vi "VI Stoermeldepuffer.vi"() -> ()   [LabVIEW 2020, in "Stoerungen.lvlib"]
uses:
  Stoerungen/Stoerungen.lvlib
  Visualisierungs Elemente/Button.ctl
  Stoerungen/FGV Stoermeldungen Aktion.ctl
  Allgemein/allgemeine Sub-VIs.lvlib
panel:
  in  "Puffer Löschen":T1
  out "Tabelle":string[][](table)
  # "Störmeldepuffer"
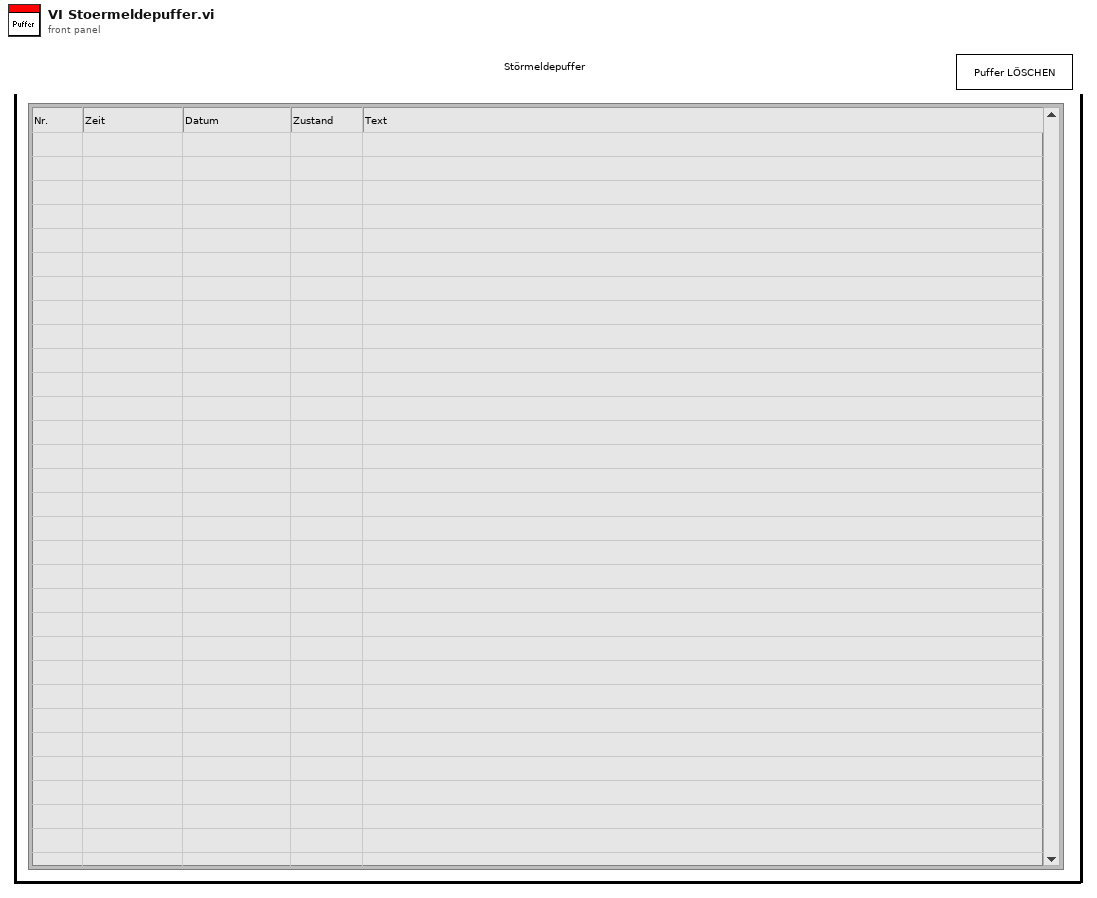
[diagram p1: front panel]
types:
  T1 = typedef "Button.ctl" = bool
  T2 = typedef "Stoerungen.lvlib/FGV Stoermeldungen Aktion.ctl" = enum16{"Initialisieren", "kommend", "gehend", "lesen", "Queue leeren", "Queue freigeben", "in Datei loggen", "Änderung zurücksetzen"}
  T3 = typedef "Stoerungen.lvlib/Stoermeldung.ctl" = cluster{"Zeitstempel":timestamp, "Nummer":i32, "Kommend":bool}
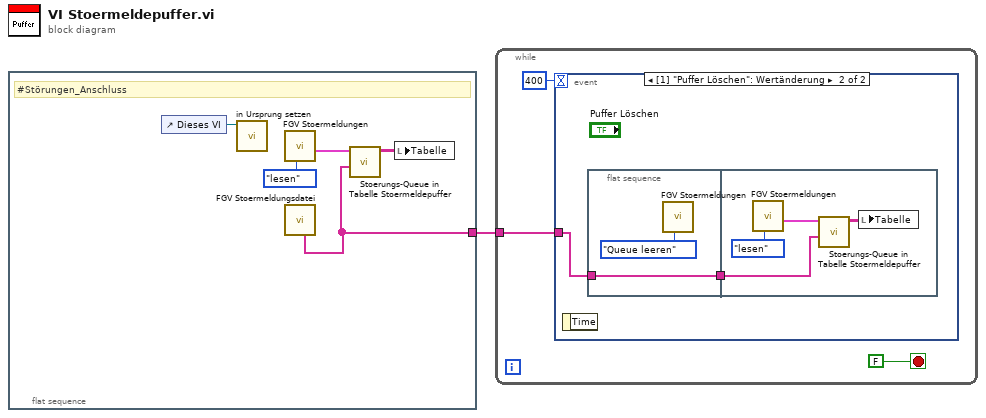
[diagram p0: block diagram]
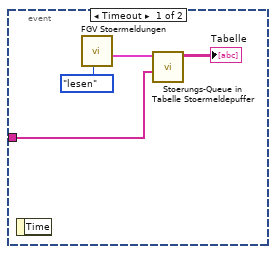
[diagram p2: hidden frame]
diagram:
  n1 = flat-sequence {
    tunnel: [w2] -> w1
    frame #0 {
      # "#Störungen_Anschluss"
      n2 = control-ref of="Dieses VI"() -> (w3:refnum<vi>)
      n3 = call "in Ursprung setzen.vi"("VI Referenz"=w3) -> ()  [unwired: 10 in, 1 out]
      n4 = call "FGV Stoermeldungen.vi"("Aktion"=FGV_Stoermeldungen_Aktion."lesen") -> ("Queue-Inhalt"=w5:T3[])  [unwired: 3 in, 7 out]
      n5 = call "FGV Stoermeldungsdatei.vi"() -> ("Text"=w2:string[])  [unwired: 3 in, 8 out]
      n6 = call "Stoerungs-Queue in Tabelle Stoermeldepuffer.vi"("Störmeldetexte aus Datei"=w2, "Queue-Inhalt (FGV Störmeldungen)"=w5) -> ("Tabelle Störmeldungen"=w4:string[][])  [unwired: 9 out]
      n7 = local write "Tabelle"(w4) -> ()
    }
  }
  n8 = while {
    tunnel: w1 -> [w8]
    stop <- FALSE stop-if-true
    n9 = event shown="[1] \"Puffer Löschen\": Wertänderung" {
      selector: _ -> [_ _]
      dyn-events: _ -> [_ _]
      timeout: 400 -> [_ _]
      tunnel: w8 -> [w10 w15]
      event Timeout {
        n10 = event-data() -> ()  [unwired: 2 out]
        n11 = call "FGV Stoermeldungen.vi"("Aktion"=FGV_Stoermeldungen_Aktion."lesen") -> ("Queue-Inhalt"=w12:T3[])  [unwired: 3 in, 7 out]
        n12 = call "Stoerungs-Queue in Tabelle Stoermeldepuffer.vi"("Störmeldetexte aus Datei"=w10, "Queue-Inhalt (FGV Störmeldungen)"=w12) -> ("Tabelle Störmeldungen"=→"Tabelle":string[][])  [unwired: 9 out]
      }
      event Value Change {
        n13 = event-data() -> ()  [unwired: 2 out]
        n14 = flat-sequence {
          tunnel: w15 -> [w16]
          tunnel: [w16] -> w14
          tunnel: w14 -> [w18]
          frame #0 {
            n15 = call "FGV Stoermeldungen.vi"("Aktion"=FGV_Stoermeldungen_Aktion."Queue leeren") -> ()  [unwired: 3 in, 8 out]
          }
          frame #1 {
            n16 = call "FGV Stoermeldungen.vi"("Aktion"=FGV_Stoermeldungen_Aktion."lesen") -> ("Queue-Inhalt"=w21:T3[])  [unwired: 3 in, 7 out]
            n17 = call "Stoerungs-Queue in Tabelle Stoermeldepuffer.vi"("Störmeldetexte aus Datei"=w18, "Queue-Inhalt (FGV Störmeldungen)"=w21) -> ("Tabelle Störmeldungen"=w19:string[][])  [unwired: 9 out]
            n18 = local write "Tabelle"(w19) -> ()
          }
        }
      }
    }
  }
